vi "task start_stop.vi"(7 "Start/Stop":enum16{"start", "stop"}(ring), 8 "Error In":errorcluster, 11 "task/channels in":refnum<k21>) -> (0 "Error Out":errorcluster, 3 "task out":refnum<k21>)   [LabVIEW 2018]
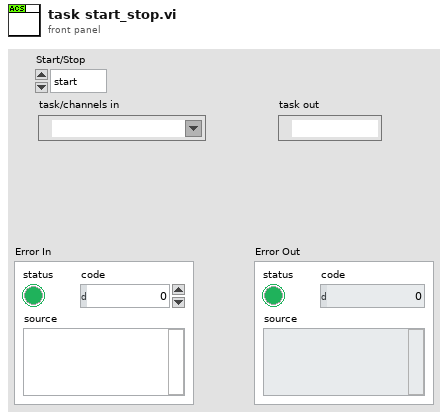
[diagram p1: front panel]
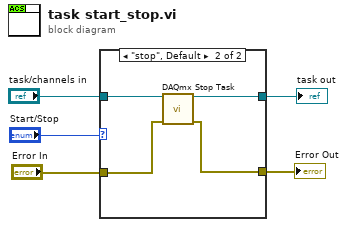
[diagram p0: block diagram]
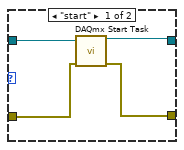
[diagram p2: hidden frame]
diagram:
  n1 = case shown="\"stop\", Default" "Start/Stop" {
    tunnel: "task/channels in" -> [w9 w13]
    tunnel: [w8 w12] -> w3
    tunnel: "Error In" -> [w7 w11]
    tunnel: [w6 w10] -> w1
    frame "start" {
      n2 = call <vilib>:"DAQmx Start Task.vi"("task/channels in"=w9, "error in"=w7) -> ("task out"=w8:refnum<k21>, "error out"=w6:errorcluster)  [unwired: 12 in]
    }
    frame "stop", Default {
      n3 = call <vilib>:"DAQmx Stop Task.vi"("task/channels in"=w13, "error in"=w11) -> ("task out"=w12:refnum<k21>, "error out"=w10:errorcluster)  [unwired: 12 in]
    }
  }
  "Error Out" <- w1
  "task out" <- w3
